vi "Erase Command.vi"(8 "error in (no error)":errorcluster, 11 "Channel in":refnum<class "Channel.lvclass">) -> (0 "error out":errorcluster, 3 "Channel out":refnum<class "Channel.lvclass">)   [LabVIEW 2018, in "Channel.lvclass"]
doc: "Erase the command received from the control interface"
uses:
  Channel.lvclass
  Channel.lvclass/Channel.ctl
  RxTx/CCS_RxTx.lvclass
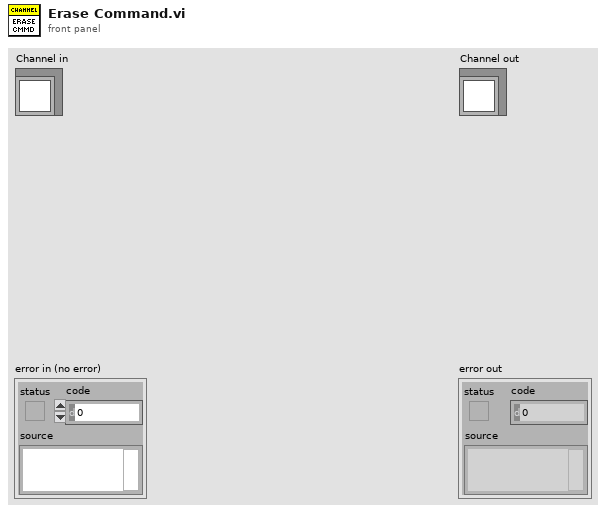
[diagram p1: front panel]
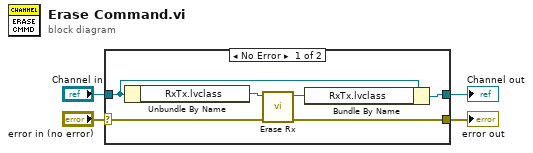
[diagram p0: block diagram]
diagram:
  n1 = case shown="No Error" "error in (no error)" {
    selector: "error in (no error)" -> [w10 w12]
    tunnel: [w9 w12] -> w3
    tunnel: [w6 w11] -> w1
    tunnel: "Channel in" -> [w7 w11]
    frame No Error {
      n2 = Unbundle By Name(w7) -> ("RxTx.lvclass"=w8:refnum<class "CCS_RxTx.lvclass">)
      n3 = call "Erase Rx.vi"("error in (no error)"=w10, "RxTx in"=w8) -> ("error out"=w9:errorcluster, "RxTx out"=w5:refnum<class "CCS_RxTx.lvclass">)  [unwired: 8 in]
      n4 = Bundle By Name(cluster=w7, "RxTx.lvclass"=w5) -> (w6:refnum<class "Channel.lvclass">)
    }
    frame Error {
    }
  }
  "error out" <- w3
  "Channel out" <- w1
